vi "Generate 4 surrounding node addresses.vi"(8 "error in (no error)":errorcluster, 11 "2D Array in":refnum<class "2D Array.lvclass">) -> (0 "error out":errorcluster, 1 "Search Directions":T1[](array[typedef])=[enum."Right", enum."Down", enum."Left", enum."Up"], 2 "4 Surrounding Nodes":refnum<class "2D Array.lvclass">[](array[class]), 3 "2D Array out":refnum<class "2D Array.lvclass">)   [LabVIEW 2019, in "2D Array.lvclass"]
uses:
  2D Array.lvclass
  Grassfire/Direction--enum.ctl
  2D Array.lvclass/2D Array.ctl
  Grassfire/Grassfire.lvclass
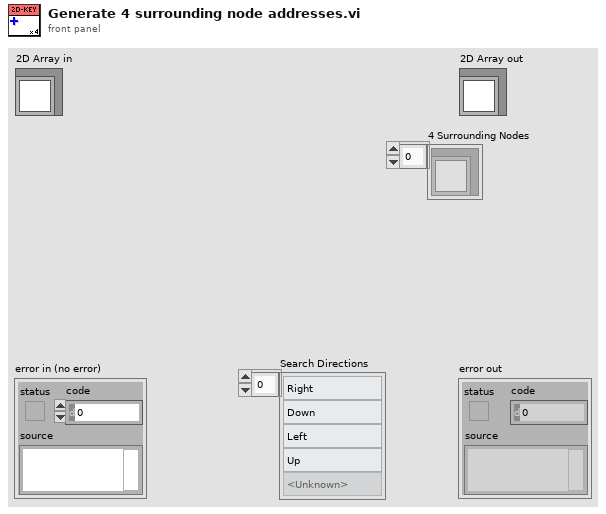
[diagram p1: front panel]
types:
  T1 = typedef "Grassfire.lvclass/Direction--enum.ctl" = enum16{"<Unknown>", "Right", "Down", "Left", "Up"}
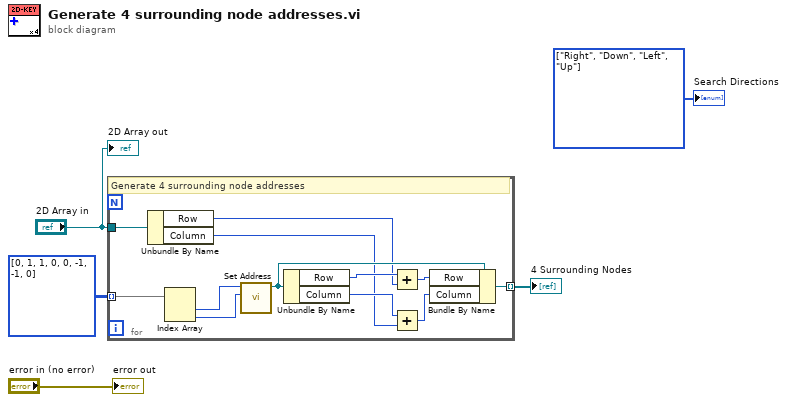
[diagram p0: block diagram]
diagram:
  w1 = T1[] [enum."Right", enum."Down", enum."Left", enum."Up"] items=["<Unknown>", "Right", "Down", "Left", "Up"]
  n1 = for {
    tunnel: i32[][] [[0, 1], [1, 0], [0, -1], [-1, 0]] -> [w17] mode=indexing
    tunnel: [w12] -> w4 mode=indexing
    tunnel: "2D Array in" -> [w14]
    # "Generate 4 surrounding node addresses"
    n2 = Unbundle By Name(w14) -> ("Row"=w10:i32, "Column"=w7:i32)
    n3 = Index Array(array=w17) -> (element #1=w16:i32, element #2=w15:i32)  [unwired: 2 in]
    n4 = call "Set Address.vi"("Column"=w15, "Row"=w16) -> ("2D Array Index"=w13:refnum<class "2D Array.lvclass">)  [unwired: 9 in]
    n5 = Unbundle By Name(w13) -> ("Row"=w11:i32, "Column"=w8:i32)
    n6 = Add(x=w11, y=w10) -> (x+y=w9:i32)
    n7 = Add(x=w8, y=w7) -> (x+y=w6:i32)
    n8 = Bundle By Name(cluster=w13, "Row"=w9, "Column"=w6) -> (w12:refnum<class "2D Array.lvclass">)
  }
  "4 Surrounding Nodes" <- w4
  "error out" <- "error in (no error)"
  "2D Array out" <- "2D Array in"
  "Search Directions" <- w1
